vi "Write INI String.vi"(6 "Force Default Session?(F)":bool, 8 "error in (no error)":errorcluster, 9 "Content":string, 10 "Variable":T1, 11 "CSM-Static-Variable-Manager in":refnum<class "CSM-Static-Variable-Manager.lvclass">) -> (0 "error out":errorcluster, 2 "Key Replaced?":bool, 3 "CSM-Static-Variable-Manager out":refnum<class "CSM-Static-Variable-Manager.lvclass">)   [LabVIEW 2017, in "INI-Static-Variable-Support.lvlib" / "CSM-Static-Variable-Manager.lvclass"]
uses:
  CSM-Static-Variable-Manager.lvclass
  _Def-Ini-Variable.ctl
  CSM-Static-Variable-Manager.lvclass/CSM-Static-Variable-Manager.ctl
  INI-Static-Variable-Support.lvlib
  LabVIEW-Config/LabVIEW-Config.lvclass
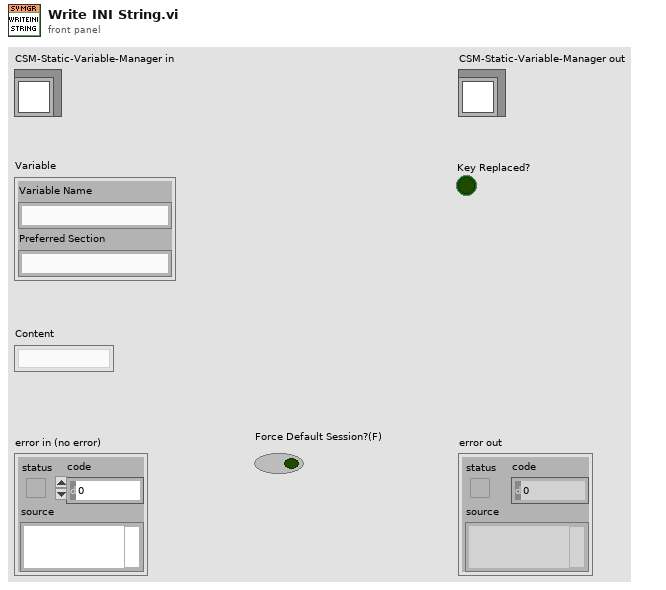
[diagram p1: front panel]
types:
  T1 = typedef "INI-Static-Variable-Support.lvlib/_Def-Ini-Variable.ctl" = cluster{"Variable Name":string, "Preferred Section":string}
  T2 = typedef "LabVIEW-Config.lvlib/Config.ctl" = cluster{"Path":path, "Lines":string[], "Tokens":T3[], "Modified?":bool, "Cache":cluster{"Valid?":bool, "Key Information":T4[]}}
  T3 = typedef "LabVIEW-Config.lvlib/LineToken.ctl" = enum8{"comment", "section", "key", "more"}
  T4 = typedef "LabVIEW-Config.lvlib/KeyInfo.ctl" = cluster{"Key Indexes":cluster{"Indexes":i32[]}[], "Session Found?":bool, "Key found?":bool, "Session Index":i32}
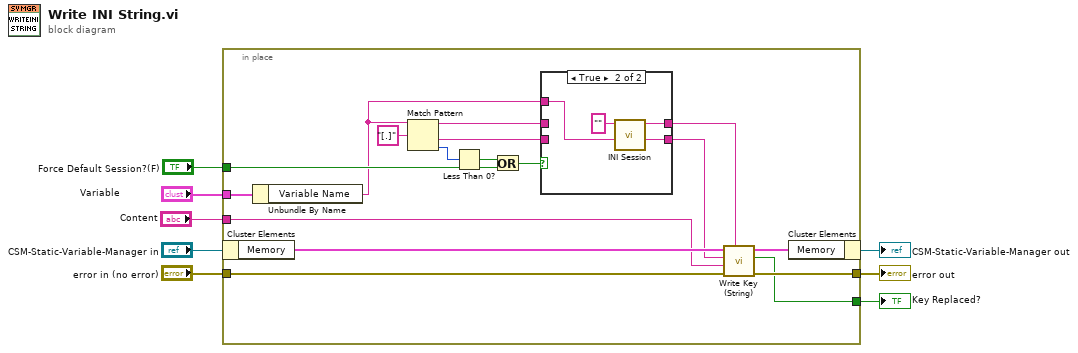
[diagram p0: block diagram]
diagram:
  n1 = in-place {
    in-place-border: "error in (no error)" -> [w23]
    in-place-border: [w22] -> w5
    in-place-border: [w21] -> w4
    in-place-border: "Variable" -> [w13]
    in-place-border: "Content" -> [w10]
    in-place-border: "Force Default Session?(F)" -> [w17]
    n2 = in-place-cluster #1("CSM-Static-Variable-Manager in") -> ("Memory"=w25:T2)
    n3 = Unbundle By Name(w13) -> ("Variable Name"=w9:string)
    n4 = Match Pattern(string=w9, regular expression="[.]") -> (before substring=w14:string, after substring=w12:string, offset past match=w19:i32)  [unwired: 1 in, 1 out]
    n5 = Less Than 0?(x=w19) -> (x < 0?=w18:bool)
    n6 = Or(x=w18, y=w17) -> (x .or. y?=w16:bool)
    n7 = case shown="True" w16 {
      tunnel: [w27 w30] -> w15
      tunnel: w14 -> [w27 _]
      tunnel: w9 -> [_ w29]
      tunnel: w12 -> [w26 _]
      tunnel: [w26 w29] -> w11
      frame False {
      }
      frame True {
        n8 = call "INI Session.vi"("Section Name(\"\" as Default)"="" ("Section Name(\"\" as Default)")) -> ("App.Name"=w30:string)  [unwired: 10 in]
      }
    }
    n9 = call "Write Key (String).vi"("Section Name"=w15, "error in (no error)"=w23, "Value"=w10, "Key Name"=w11, "Config in"=w25) -> ("error out"=w22:errorcluster, "Key Replaced?"=w21:bool, "Config out"=w24:T2)  [unwired: 4 in]
    n10 = in-place-cluster #1("Memory"=w24) -> (→"CSM-Static-Variable-Manager out":refnum<class "CSM-Static-Variable-Manager.lvclass">)
  }
  "error out" <- w5
  "Key Replaced?" <- w4
